vi "Res Mirror Amplitude to Trigger Delay.vi"(1 "Amplitude (V)":dbl) -> (0 "Trigger Delay (Ticks)":u16)   [LabVIEW 2014]
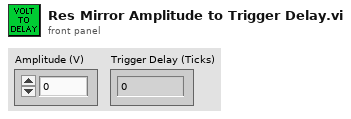
[diagram p1: front panel]
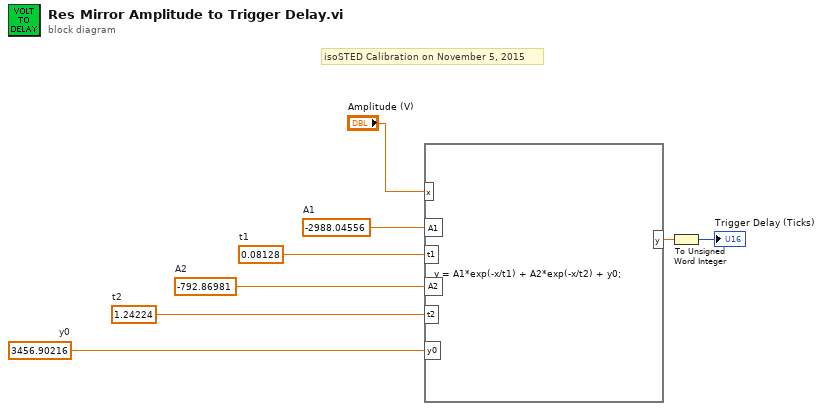
[diagram p0: block diagram]
diagram:
  w1 = 3456.90216  # y0
  w5 = 1.24224  # t2
  w6 = -792.86981  # A2
  w7 = 0.08128  # t1
  w8 = -2988.04556  # A1
  # "isoSTED Calibration on November 5, 2015"
  n1 = formula code="y = A1*exp(-x/t1) + A2*exp(-x/t2) + y0;"("A1"=w8, "t1"=w7, "A2"=w6, "t2"=w5, "x"="Amplitude (V)", "y0"=w1) -> ("y"=w3:dbl)
  n2 = To Unsigned Word Integer(number=w3) -> (unsigned 16bit integer=→"Trigger Delay (Ticks)":u16)
